vi "Generate Single Pulse.vi"   [LabVIEW 2015]
uses:
  <vilib>/DAQmx/write.llb/DAQmx Write (Digital Bool 1Line 1Point).vi
  <vilib>/DAQmx/create/channels.llb/DAQmx Create Channel (DO-Digital Output).vi
  <vilib>/DAQmx/miscellaneous.llb/DAQmx Fill In Error Info.vi
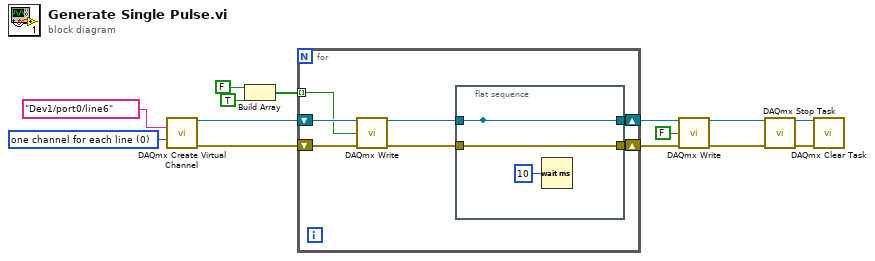
[diagram p0: block diagram]
diagram:
  w13 = 0 items=["one channel for each line", "one channel for all lines"] ("line grouping")
  n1 = call-poly <vilib>:"DAQmx Create Virtual Channel.vi"("lines"=tag "Dev1/port0/line6", "line grouping"=w13) -> ("task out"=w12:refnum<k21>, "error out"=w11:errorcluster)  [unwired: 12 in]
  n2 = Build Array(FALSE, TRUE ("element")) -> (w1:bool[])
  n3 = for {
    shift-right: [w16] -> w8
    shift-left: w12 -> [w21]
    shift-right: [w17] -> w9
    shift-left: w11 -> [w20]
    tunnel: w1 -> [w15] mode=indexing
    n4 = call-poly <vilib>:"DAQmx Write.vi"("task/channels in"=w21, "data"=w15, "error in"=w20) -> ("task out"=w19:refnum<k21>, "error out"=w18:errorcluster)  [unwired: 10 in, 1 out]
    n5 = flat-sequence {
      tunnel: w19 -> [w22]
      tunnel: w18 -> [w23]
      tunnel: [w22] -> _
      tunnel: [w23] -> w17
      tunnel: [w22] -> w16
      frame #0 {
        n6 = Wait (ms)(milliseconds to wait=u32 10) -> ()  [unwired: 1 out]
      }
    }
  }
  n7 = call-poly <vilib>:"DAQmx Write.vi"("task/channels in"=w8, "data"=FALSE, "error in"=w9) -> ("task out"=w6:refnum<k21>, "error out"=w7:errorcluster)  [unwired: 10 in, 1 out]
  n8 = call <vilib>:"DAQmx Stop Task.vi"("task/channels in"=w6, "error in"=w7) -> ("task out"=w5:refnum<k21>, "error out"=w4:errorcluster)  [unwired: 12 in]
  n9 = call <vilib>:"DAQmx Clear Task.vi"("task in"=w5, "error in"=w4) -> ()  [unwired: 13 in, 1 out]
